vi "Teleop.vi"(10 "Match Info":T1={"Autonomous Elapsed Seconds"=0.0, "TeleOp Elapsed Seconds"=0.0, "Disabled Elapsed Seconds"=0.0, "Visited Autonomous"=FALSE, "Visited TeleOp"=FALSE, "Visited Disabled"=FALSE, "Autonomous Settings"={"Autonomous Style"=enum."Independent", "VI Refnum"=refnum}}, 11 "Call Context":T2) -> ()   [LabVIEW 2018]
doc: "This VI is called for each TeleOp packet received from the DS where the robot is not disabled. It is often used to read from the joysticks and update I/O or to update setpoints for timed control loops. It should complete and return within 20 milliseconds or it may miss DS packets."
uses:
  <vilib>/Rock Robotics/WPI/DriverStation/WPI_DriverStationDerivedRobotMode.ctl
  <vilib>/Rock Robotics/WPI/DriverStation/WPI_DriverStationMatch Info.ctl
  <vilib>/Rock Robotics/WPI/ThirdParty/Phoenix-LabVIEW/Motor Controller/Controls/CTRE_Phoenix_MotorControl_ControlMode.ctl
  <vilib>/Rock Robotics/WPI/Solenoid/WPI_SolenoidValue.ctl
  <vilib>/Rock Robotics/WPI/Utilities/WPI_GetSetVariantRefNum.vi
  <vilib>/Rock Robotics/Network Tables/NT Write Boolean Array.vi
  <vilib>/Rock Robotics/Network Tables/NT Write Numeric Array.vi
  <vilib>/Rock Robotics/WPI/Solenoid/WPI_SolenoidSetEnum.vi
  Global 1.vi
panel:
  # "r"
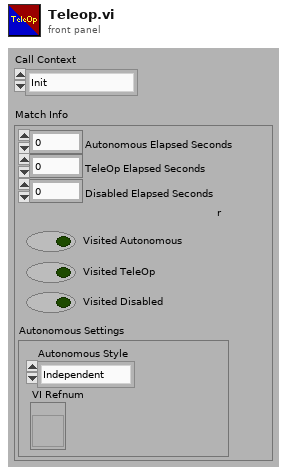
[diagram p1: front panel]
types:
  T1 = typedef "WPI_DriverStationMatch Info.ctl" = cluster{"Autonomous Elapsed Seconds":dbl, "TeleOp Elapsed Seconds":dbl, "Disabled Elapsed Seconds":dbl, "Visited Autonomous":bool, "Visited TeleOp":bool, "Visited Disabled":bool, "Autonomous Settings":cluster{"Autonomous Style":enum16{"Iterative", "Independent"}, "VI Refnum":refnum<vi>}}
  T2 = typedef "WPI_DriverStationDerivedRobotMode.ctl" = enum16{"Init", "Execute", "Stop"}
  T3 = typedef "WPI_JoystickDevRef.ctl" = cluster{"Device":T4}
  T4 = typedef "WPI_JoystickDeviceEnum.ctl" = enum16{"USB 0", "USB 1", "USB 2", "USB 3", "USB 4", "USB 5"}
  T5 = typedef "WPI_SwitchDevRef.ctl" = cluster{"DevStatus":errorcluster, "DIO Channel":T6, "CntIndex":T7, "Normally Closed":bool}
  T6 = typedef "FPGA_DIOChannel.ctl" = enum8{"DIO 0", "DIO 1", "DIO 2", "DIO 3", "DIO 4", "DIO 5", "DIO 6", "DIO 7", "DIO 8", "DIO 9", "DIO MXP 0", "DIO MXP 1", "DIO MXP 2", "DIO MXP 3", "DIO MXP 4", "DIO MXP 5", "DIO MXP 6", "DIO MXP 7", "DIO MXP 8", "DIO MXP 9", "DIO MXP 10", "DIO MXP 11", "DIO MXP 12", "DIO MXP 13", "DIO MXP 14", "DIO MXP 15", "SPI Port CS1", "SPI Port CS2", "SPI Port CS3", "SPI Port MISO", "SPI Port MOSI", "Invalid"}
  T7 = typedef "FPGA_CounterCtrSystemIndex.ctl" = enum8{"Ctr 0", "Ctr 1", "Ctr 2", "Ctr 3", "Ctr 4", "Ctr 5", "Ctr 6", "Ctr 7", "Invalid"}
  T8 = typedef "WPI_SolenoidDevRef.ctl" = cluster{"DevStatus":errorcluster, "Pneumatics Control Module":u8, "Forward Solenoid Channel":T9, "Reverse Solenoid Channel":T9}
  T9 = typedef "WPI_SolenoidChannel.ctl" = enum8{"Solenoid 0", "Solenoid 1", "Solenoid 2", "Solenoid 3", "Solenoid 4", "Solenoid 5", "Solenoid 6", "Solenoid 7", "Invalid"}
  T10 = typedef "WPI_MotorControlDeviceRef.ctl" = cluster{"DeviceStatus":errorcluster, "Type":T11, "PWM":cluster{"PWM Channel":T12, "DeadBand":T13}, "CAN":cluster{"Device Number":u8, "SetOutput VI Ref":variant, "GetOutput VI Ref":variant, "Enable VI Ref":variant, "Disable VI Ref":variant, "Data":variant}, "Invert":bool, "DIO PWM":cluster{"PWM \"Enable\" Channel":T12, "DIOChannel":T6, "PWM Rate":dbl}}
  T11 = typedef "WPI_MotorControlType.ctl" = enum16{"PWM", "CAN", "DIO PWM"}
  T12 = typedef "FPGA_DIOPWMChannel.ctl" = enum8{"PWM 0", "PWM 1", "PWM 2", "PWM 3", "PWM 4", "PWM 5", "PWM 6", "PWM 7", "PWM 8", "PWM 9", "PWM MXP 0", "PWM MXP 1", "PWM MXP 2", "PWM MXP 3", "PWM MXP 4", "PWM MXP 5", "PWM MXP 6", "PWM MXP 7", "PWM MXP 8", "PWM MXP 9", "Invalid"}
  T13 = typedef "WPI_PWMDeadband.ctl" = cluster{"Name":string, "maxPositivePwm":i32, "minPositivePwm":i32, "centerPwm":i32, "maxNegativePwm":i32, "minNegativePwm":i32, "angularRange":u16}
  T14 = typedef "CTRE_Phoenix_MotorControl_ControlMode.ctl" = u16
  T15 = typedef "WPI_SolenoidValue.ctl" = enum16{"Off", "On", "Forward", "Reverse"}
  T16 = typedef "WPI_RobotDriveDevRef.ctl" = cluster{"DevStatus":errorcluster, "Motors[]":T10[], "Square Inputs":bool, "Max Output":dbl}
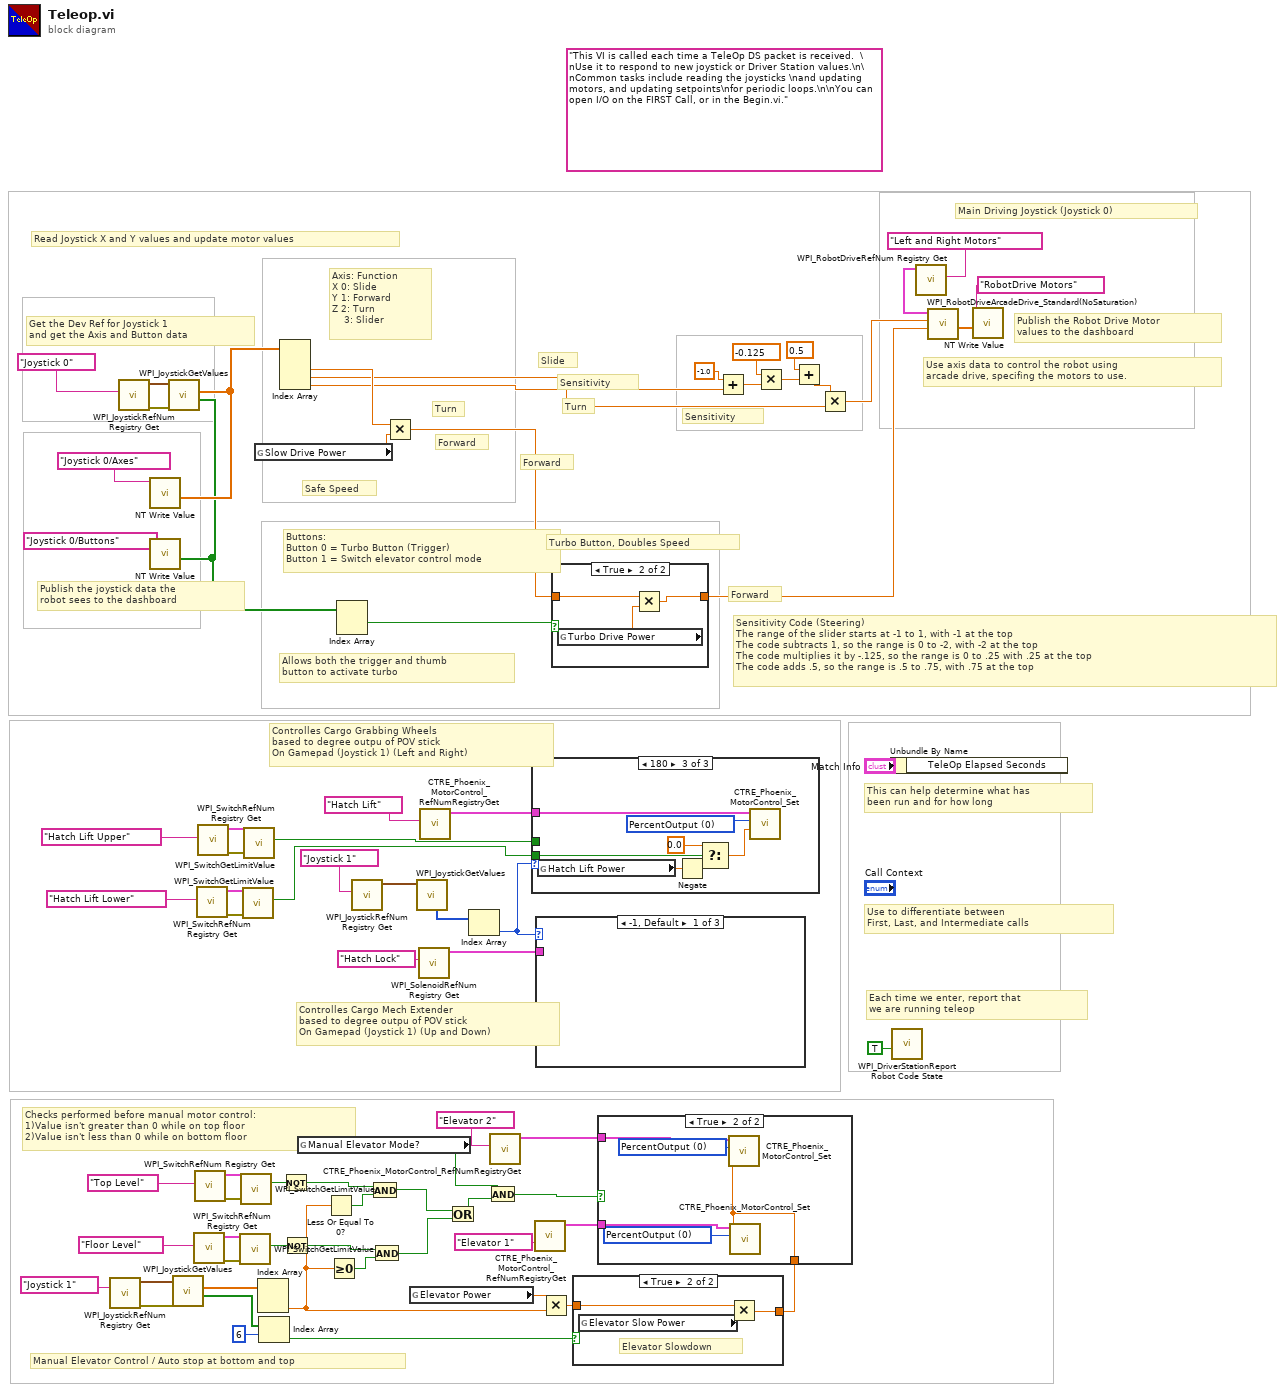
[diagram p0: block diagram]
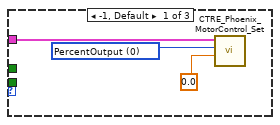
[diagram p2: hidden frame]
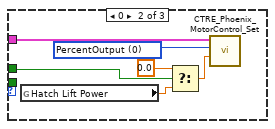
[diagram p3: hidden frame]
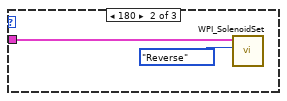
[diagram p4: hidden frame]
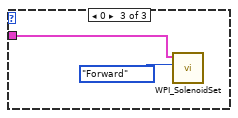
[diagram p5: hidden frame]
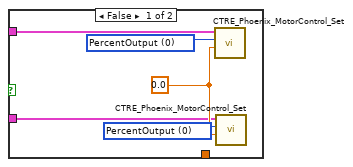
[diagram p7: hidden frame]
diagram:
  (unwired) "This VI is called each time a TeleOp DS packet is received.  \nUse it to respond to new joystick or Driver Station values.\n\nCommon tasks include reading the joysticks \nand updating motors, and updating setpoints\nfor periodic loops.\n\nYou can open I/O on the FIRST Call, or in the Begin.vi."
  # "Controlles Cargo Mech Extender \nbased to degree outpu of POV stick\nOn Gamepad (Joystick 1) (Up and Down)"
  # "Controlles Cargo Grabbing Wheels \nbased to degree outpu of POV stick\nOn Gamepad (Joystick 1) (Left and Right)"
  # "Checks performed before manual motor control:\n1)Value isn't greater than 0 while on top floor\n2)Value isn't less than 0 while on bottom floor"
  # "Manual Elevator Control / Auto stop at bottom and top"
  # "Sensitivity Code (Steering)\nThe range of the slider starts at -1 to 1, with -1 at the top\nThe code subtracts 1, so the range is 0 to -2, with -2 at the top\nThe code multiplies it by -.125, so the range is 0 to .25 with .25 at the top\nThe code adds .5, so the range is .5 to .75, with .75 at the top"
  # "Sensitivity"
  # "Sensitivity"
  # "Allows both the trigger and thumb\nbutton to activate turbo"
  # "Slide"
  # "Use axis data to control the robot using\narcade drive, specifing the motors to use."
  # "Get the Dev Ref for Joystick 1\nand get the Axis and Button data"
  # "Turn"
  # "Forward"
  # "Forward"
  # "Main Driving Joystick (Joystick 0)"
  # "Buttons:\nButton 0 = Turbo Button (Trigger)\nButton 1 = Switch elevator control mode"
  # "Safe Speed"
  # "Turbo Button, Doubles Speed"
  # "Forward"
  # "Turn"
  # "Axis: Function\nX 0: Slide \nY 1: Forward\nZ 2: Turn\n    3: Slider"
  # "Publish the Robot Drive Motor\nvalues to the dashboard"
  # "Publish the joystick data the\nrobot sees to the dashboard"
  # "Read Joystick X and Y values and update motor values"
  # "Each time we enter, report that\nwe are running teleop"
  # "Use to differentiate between\nFirst, Last, and Intermediate calls"
  # "This can help determine what has\nbeen run and for how long"
  n1 = call <vilib>:"WPI_JoystickRefNum Registry Get.vi"("refnum name"="Joystick 1") -> ("error out"=w9:errorcluster, "JoystickDevRef"=w44:T3)  [unwired: 1 in, 8 out]
  n2 = call <vilib>:"WPI_JoystickRefNum Registry Get.vi"("refnum name"="Joystick 0") -> ("error out"=w13:errorcluster, "JoystickDevRef"=w70:T3)  [unwired: 1 in, 8 out]
  n3 = call <vilib>:"WPI_JoystickGetValues.vi"("error in (no error)"=w13, "JoystickDevRef"=w70) -> ("Buttons"=w62:bool[], "Axes"=w67:dbl[])  [unwired: 5 in, 3 out]
  n4 = call-poly <vilib>:"NT Write Value.vi"("Numeric Array"=w67, "Name"="Joystick 0/Axes") -> ()  [unwired: 9 in, 1 out]
  n5 = call-poly <vilib>:"NT Write Value.vi"("Boolean Array"=w62, "Name"="Joystick 0/Buttons") -> ()  [unwired: 9 in, 1 out]
  n6 = call <vilib>:"WPI_JoystickGetValues.vi"("error in (no error)"=w9, "JoystickDevRef"=w44) -> ("Buttons"=w26:bool[], "Axes"=w49:dbl[])  [unwired: 5 in, 3 out]
  n7 = call <vilib>:"WPI_SwitchRefNum Registry Get.vi"("refnum name"="Floor Level") -> ("error out"=w10:errorcluster, "SwitchDevRef"=w53:T5)  [unwired: 9 in]
  n8 = call <vilib>:"WPI_SwitchRefNum Registry Get.vi"("refnum name"="Top Level") -> ("error out"=w11:errorcluster, "SwitchDevRef"=w52:T5)  [unwired: 9 in]
  n9 = call <vilib>:"WPI_SwitchRefNum Registry Get.vi"("refnum name"="Hatch Lift Lower") -> ("error out"=w3:errorcluster, "SwitchDevRef"=w6:T5)  [unwired: 9 in]
  n10 = call <vilib>:"WPI_SwitchRefNum Registry Get.vi"("refnum name"="Hatch Lift Upper") -> ("error out"=w4:errorcluster, "SwitchDevRef"=w5:T5)  [unwired: 9 in]
  n11 = call <vilib>:"WPI_SwitchGetLimitValue.vi"("error in (no error)"=w10, "SwitchDevRef"=w53) -> ("Switch Pressed"=w51:bool)  [unwired: 7 in, 2 out]
  n12 = call <vilib>:"WPI_SwitchGetLimitValue.vi"("error in (no error)"=w11, "SwitchDevRef"=w52) -> ("Switch Pressed"=w50:bool)  [unwired: 7 in, 2 out]
  n13 = call <vilib>:"WPI_SwitchGetLimitValue.vi"("error in (no error)"=w3, "SwitchDevRef"=w6) -> ("Switch Pressed"=w2:bool)  [unwired: 7 in, 2 out]
  n14 = call <vilib>:"WPI_SwitchGetLimitValue.vi"("error in (no error)"=w4, "SwitchDevRef"=w5) -> ("Switch Pressed"=w1:bool)  [unwired: 7 in, 2 out]
  n15 = global read "Global 1.vi" "Slow Drive Power"() -> (w57:dbl)
  n16 = Index Array(array=w49) -> (element #2=w31:dbl)  [unwired: 2 in, 1 out]
  n17 = Index Array(array=w26, index=6) -> (element=w24:bool)
  n18 = Index Array(array=w67) -> (element #2=w63:dbl, element #3=w60:dbl, element #4=w59:dbl)  [unwired: 4 in, 1 out]
  n19 = Not(x=w50) -> (.not. x?=w40:bool)
  n20 = Not(x=w51) -> (.not. x?=w39:bool)
  n21 = global read "Global 1.vi" "Manual Elevator Mode?"() -> (w43:bool)
  n22 = Less Or Equal To 0?(x=w31) -> (x <= 0?=w42:bool)
  n23 = Greater Or Equal To 0?(x=w31) -> (x >= 0?=w41:bool)
  n24 = Index Array(array=w62) -> (element #1=w56:bool)  [unwired: 2 in, 1 out]
  n25 = call <vilib>:"WPI_JoystickRefNum Registry Get.vi"("refnum name"="Joystick 1") -> ("JoystickDevRef"=w22:T3)  [unwired: 1 in, 9 out]
  n26 = And(x=w40, y=w42) -> (x .and. y?=w35:bool)
  n27 = And(x=w39, y=w41) -> (x .and. y?=w32:bool)
  n28 = Multiply(x=w63, y=w57) -> (x*y=w64:dbl)
  n29 = global read "Global 1.vi" "Elevator Power"() -> (w46:dbl)
  n30 = call <vilib>:"WPI_JoystickGetValues.vi"("JoystickDevRef"=w22) -> ("POVs"=w21:i16[])  [unwired: 6 in, 4 out]
  n31 = call <vilib>:"WPI_SolenoidRefNum Registry Get.vi"("refnum name"="Hatch Lock") -> ("SolenoidDevRef"=w17:T8)  [unwired: 9 in, 1 out]
  n32 = call <vilib>:"CTRE_Phoenix_MotorControl_RefNumRegistryGet.vi"("refnum name"="Hatch Lift") -> ("PhoenixMotorControlDevRef"=w12:T10)  [unwired: 9 in, 1 out]
  n33 = Or(x=w35, y=w32) -> (x .or. y?=w33:bool)
  n34 = Index Array(array=w21) -> (element=w18:i16)  [unwired: 1 in]
  n35 = And(x=w43, y=w33) -> (x .and. y?=w34:bool)
  n36 = call <vilib>:"CTRE_Phoenix_MotorControl_RefNumRegistryGet.vi"("refnum name"="Elevator 2") -> ("PhoenixMotorControlDevRef"=w29:T10)  [unwired: 9 in, 1 out]
  n37 = case shown="180" w18 {
    tunnel: w12 -> [w78 w83 w91]
    tunnel: w2 -> [_ _ w85]
    tunnel: w1 -> [_ w79 _]
    frame -1, Default {
      w77 = T14 0 items=["PercentOutput"=0, "Position"=1, "Velocity"=2, "Current"=3, "Follower"=5, "MotionProfile"=6, "MotionMagic"=7, "MotionProfileArc"=10, "Disabled"=15] ("Control Mode")
      n38 = call <vilib>:"CTRE_Phoenix_MotorControl_Set.vi"("Output"=0.0, "Control Mode"=w77, "PhoenixMotorControlDevRef"=w78) -> ()  [unwired: 7 in, 2 out]
    }
    frame 0 {
      w84 = T14 0 items=["PercentOutput"=0, "Position"=1, "Velocity"=2, "Current"=3, "Follower"=5, "MotionProfile"=6, "MotionMagic"=7, "MotionProfileArc"=10, "Disabled"=15] ("Control Mode")
      n39 = global read "Global 1.vi" "Hatch Lift Power"() -> (w82:dbl)
      n40 = Select(t=0.0, s=w79, f=w82) -> (s? t:f=w81:dbl)
      n41 = call <vilib>:"CTRE_Phoenix_MotorControl_Set.vi"("Output"=w81, "Control Mode"=w84, "PhoenixMotorControlDevRef"=w83) -> ()  [unwired: 7 in, 2 out]
    }
    frame 180 {
      w90 = T14 0 items=["PercentOutput"=0, "Position"=1, "Velocity"=2, "Current"=3, "Follower"=5, "MotionProfile"=6, "MotionMagic"=7, "MotionProfileArc"=10, "Disabled"=15] ("Control Mode")
      n42 = global read "Global 1.vi" "Hatch Lift Power"() -> (w89:dbl)
      n43 = Negate(x=w89) -> (-x=w86:dbl)
      n44 = Select(t=0.0, s=w85, f=w86) -> (s? t:f=w87:dbl)
      n45 = call <vilib>:"CTRE_Phoenix_MotorControl_Set.vi"("Output"=w87, "Control Mode"=w90, "PhoenixMotorControlDevRef"=w91) -> ()  [unwired: 7 in, 2 out]
    }
  }
  n46 = call <vilib>:"CTRE_Phoenix_MotorControl_RefNumRegistryGet.vi"("refnum name"="Elevator 1") -> ("PhoenixMotorControlDevRef"=w47:T10)  [unwired: 9 in, 1 out]
  n47 = case shown="-1, Default" w18 {
    tunnel: w17 -> [_ w93 w94]
    frame -1, Default {
    }
    frame 180 {
      n48 = call-poly <vilib>:"WPI_SolenoidSet.vi"("Value"=WPI_SolenoidValue."Reverse", "SolenoidDevRef"=w93) -> ()  [unwired: 8 in, 2 out]
    }
    frame 0 {
      n49 = call-poly <vilib>:"WPI_SolenoidSet.vi"("Value"=WPI_SolenoidValue."Forward", "SolenoidDevRef"=w94) -> ()  [unwired: 8 in, 2 out]
    }
  }
  n50 = Multiply(x=w46, y=w31) -> (x*y=w27:dbl)
  n51 = case shown="True" w56 {
    tunnel: w64 -> [w96 w99]
    tunnel: [w96 w98] -> w16
    frame False {
    }
    frame True {
      n52 = global read "Global 1.vi" "Turbo Drive Power"() -> (w97:dbl)
      n53 = Multiply(x=w99, y=w97) -> (x*y=w98:dbl)
    }
  }
  n54 = case shown="True" w24 {
    tunnel: [w100 w102] -> w28
    tunnel: w27 -> [w100 w103]
    frame False {
    }
    frame True {
      # "Elevator Slowdown"
      n55 = global read "Global 1.vi" "Elevator Slow Power"() -> (w101:dbl)
      n56 = Multiply(x=w103, y=w101) -> (x*y=w102:dbl)
    }
  }
  n57 = case shown="True" w34 {
    tunnel: w28 -> [_ w110]
    tunnel: w47 -> [w104 w112]
    tunnel: w29 -> [w105 w111]
    frame False {
      w106 = 0.0
      w107 = T14 0 items=["PercentOutput"=0, "Position"=1, "Velocity"=2, "Current"=3, "Follower"=5, "MotionProfile"=6, "MotionMagic"=7, "MotionProfileArc"=10, "Disabled"=15] ("Control Mode")
      w108 = T14 0 items=["PercentOutput"=0, "Position"=1, "Velocity"=2, "Current"=3, "Follower"=5, "MotionProfile"=6, "MotionMagic"=7, "MotionProfileArc"=10, "Disabled"=15] ("Control Mode")
      n58 = call <vilib>:"CTRE_Phoenix_MotorControl_Set.vi"("Output"=w106, "Control Mode"=w107, "PhoenixMotorControlDevRef"=w105) -> ()  [unwired: 7 in, 2 out]
      n59 = call <vilib>:"CTRE_Phoenix_MotorControl_Set.vi"("Output"=w106, "Control Mode"=w108, "PhoenixMotorControlDevRef"=w104) -> ()  [unwired: 7 in, 2 out]
    }
    frame True {
      w109 = T14 0 items=["PercentOutput"=0, "Position"=1, "Velocity"=2, "Current"=3, "Follower"=5, "MotionProfile"=6, "MotionMagic"=7, "MotionProfileArc"=10, "Disabled"=15] ("Control Mode")
      w113 = T14 0 items=["PercentOutput"=0, "Position"=1, "Velocity"=2, "Current"=3, "Follower"=5, "MotionProfile"=6, "MotionMagic"=7, "MotionProfileArc"=10, "Disabled"=15] ("Control Mode")
      n60 = call <vilib>:"CTRE_Phoenix_MotorControl_Set.vi"("Output"=w110, "Control Mode"=w109, "PhoenixMotorControlDevRef"=w111) -> ()  [unwired: 7 in, 2 out]
      n61 = call <vilib>:"CTRE_Phoenix_MotorControl_Set.vi"("Output"=w110, "Control Mode"=w113, "PhoenixMotorControlDevRef"=w112) -> ()  [unwired: 7 in, 2 out]
    }
  }
  n62 = Add(x=-1.0, y=w59) -> (x+y=w14:dbl)
  n63 = Multiply(x=-0.125 ("y"), y=w14) -> (x*y=w37:dbl)
  n64 = Add(x=0.5, y=w37) -> (x+y=w38:dbl)
  n65 = Multiply(x=w38, y=w60) -> (x*y=w58:dbl)
  n66 = Unbundle By Name("Match Info") -> ()  [unwired: 1 out]
  n67 = call <vilib>:"WPI_DriverStationReport Robot Code State.vi"("TeleOp"=TRUE ("Autonomous")) -> ()  [unwired: 10 in, 1 out]
  n68 = call <vilib>:"WPI_RobotDriveRefNum Registry Get.vi"("refnum name"="Left and Right Motors") -> ("RobotDriveDevRef"=w72:T16)  [unwired: 1 in, 9 out]
  n69 = call <vilib>:"WPI_RobotDriveArcadeDrive_Standard(NoSaturation).vi"("Y axis value"=w16, "X axis value"=w58, "RobotDriveDevRef"=w72) -> ("Motor Values"=w66:dbl[])  [unwired: 1 in, 7 out]
  n70 = call-poly <vilib>:"NT Write Value.vi"("Numeric Array"=w66, "Name"="RobotDrive Motors") -> ()  [unwired: 9 in, 1 out]
